vi "microplastic classifier front end.vi"() -> ()   [LabVIEW 2020]
panel:
  out "found processed and matched experimental data":bool
  out "Python Backend Log":string
  out "found mp library pickle":bool
  out "found python module":bool
  in  "Tab Control":enum32{"Experiment", "Library / Admin"}(tab)
  out "library entries":dbl
  out "Library Loaded":bool
  out "Min":dbl
  out "Max":dbl
  in  "Experimental Data Path":path=path "C:/Users/Matt/Desktop/Complete Lab View Programs/Microplastic Classifier V3/experimental data"
  in  "load  process match pickle exp data":bool
  in  "Export csv":bool
  in  "Export Images":bool
  in  "refresh library info":bool
  out "Boolean":bool
  out "saving pickle":bool
  in  "create pickle file from library":bool
  in  "error in (no error)":errorcluster
  out "error out 2":errorcluster
  in  "Raw Library Path":path=path "C:/Users/Matt/Desktop/Complete Lab View Programs/Microplastic Classifier V3/mp library"
  out "saved pickle":bool
  out "return value":i32
  in  "add test":bool
  in  "return path test":bool
  out "retunr path":string
  out "String":string
  out "Numeric":i32
  out "Numeric 2":i32
  out "Instructions":string
  in  "stop":bool
  # "Import Experimental Data\n    Step 1: Drag Experimental Data Folder into the box below\n    Step 2: Click the button to Load, Process & Match Data"
  # "Generate Reports:\n    -Step 3. Export .csv file or Export spectra images"
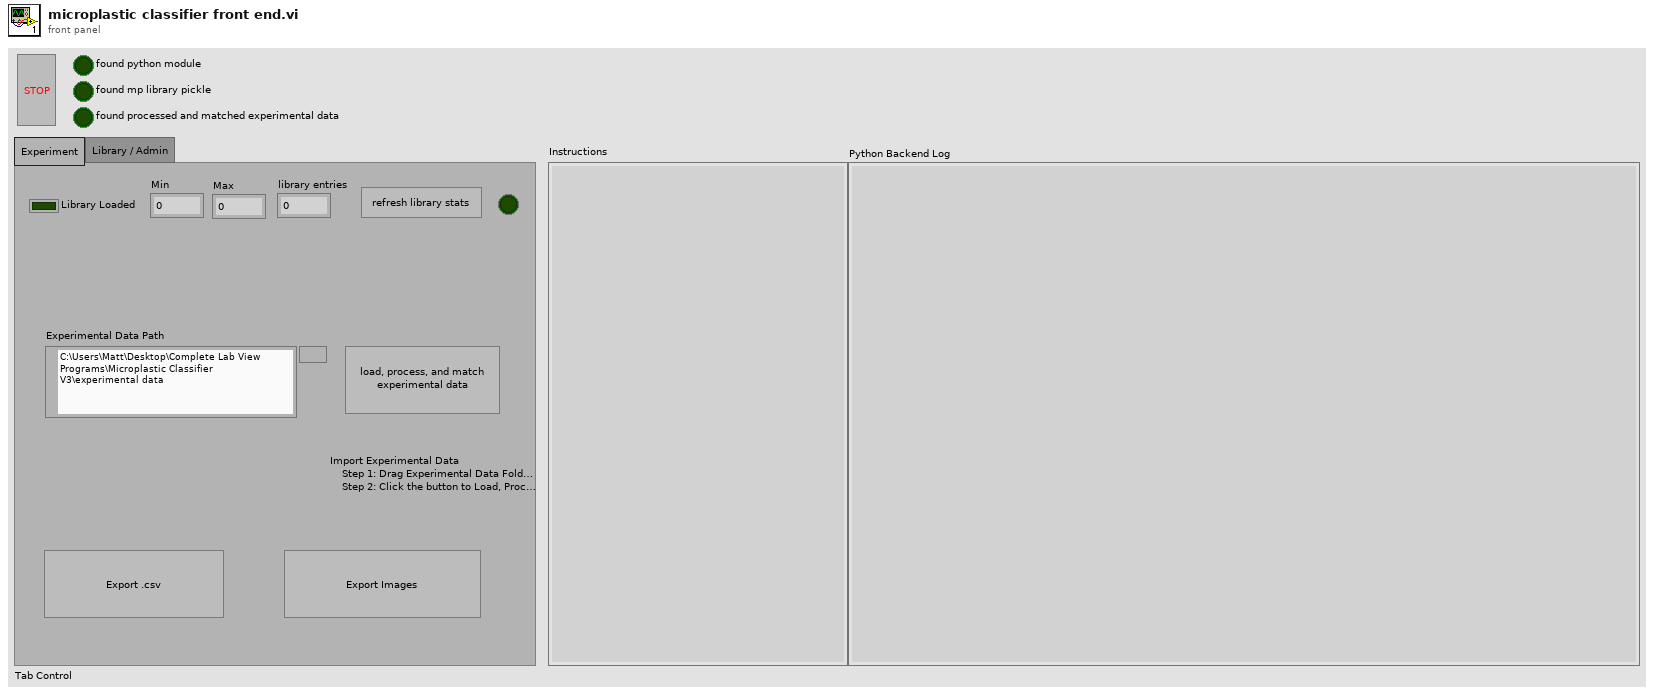
[diagram p1: front panel]
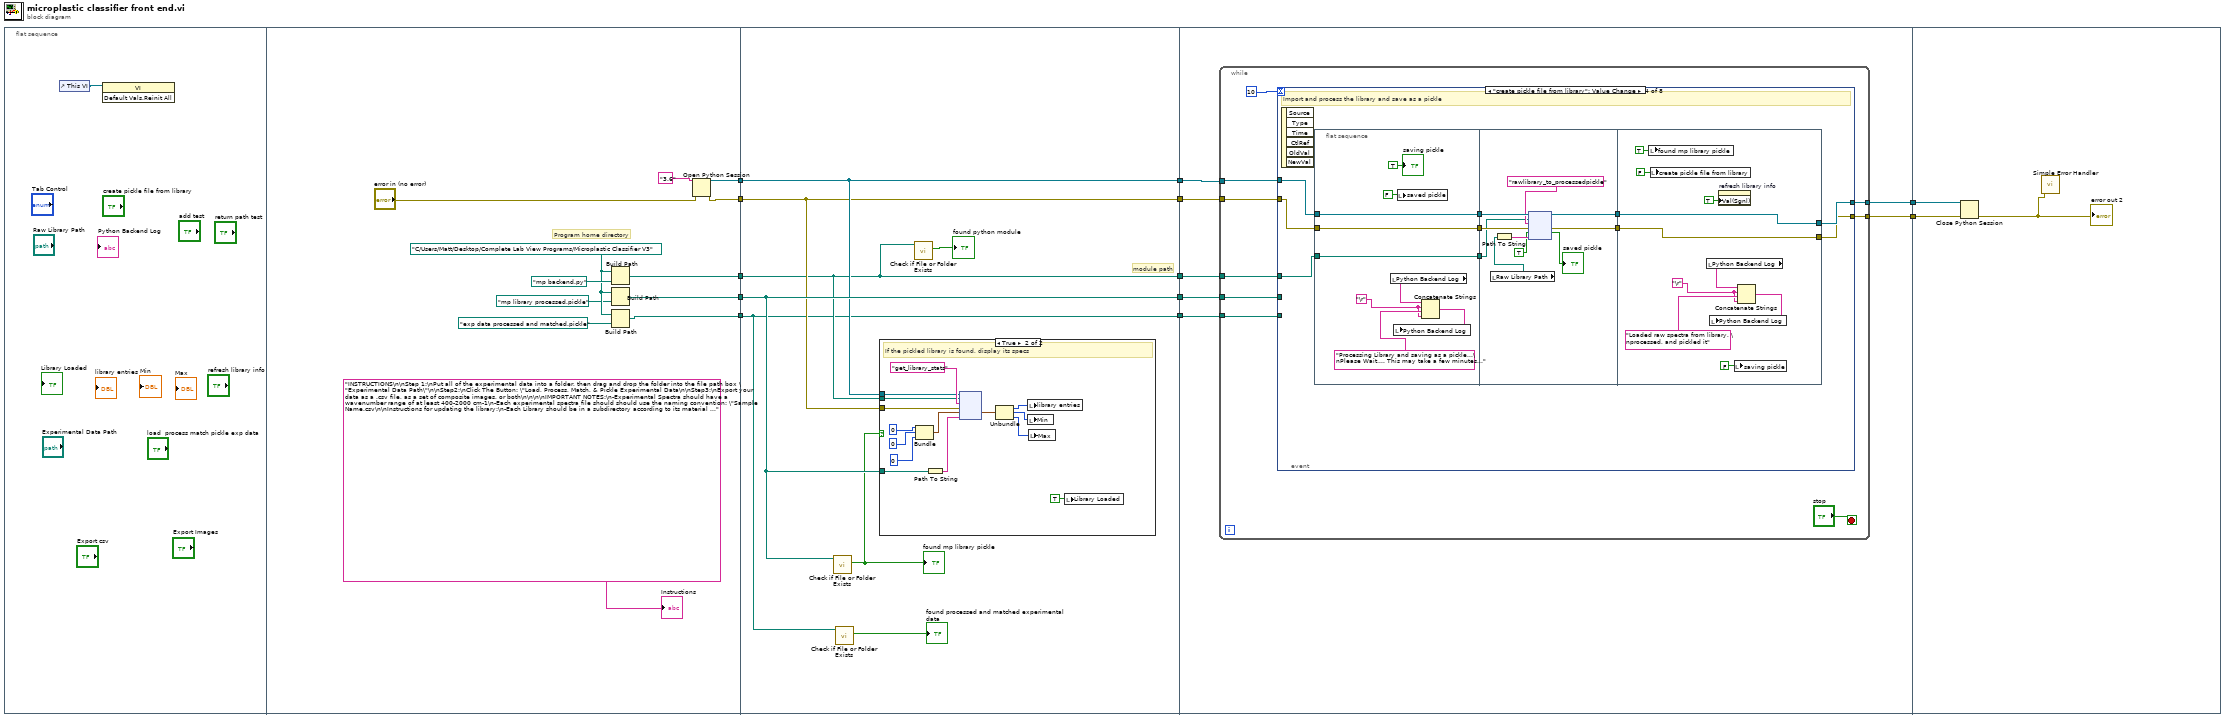
[diagram p0: block diagram]
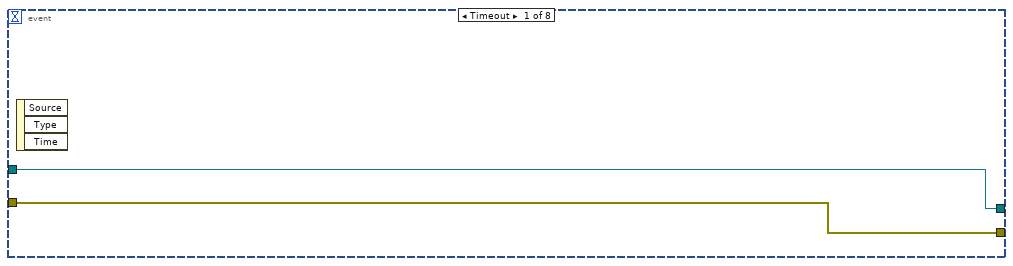
[diagram p3: hidden frame]
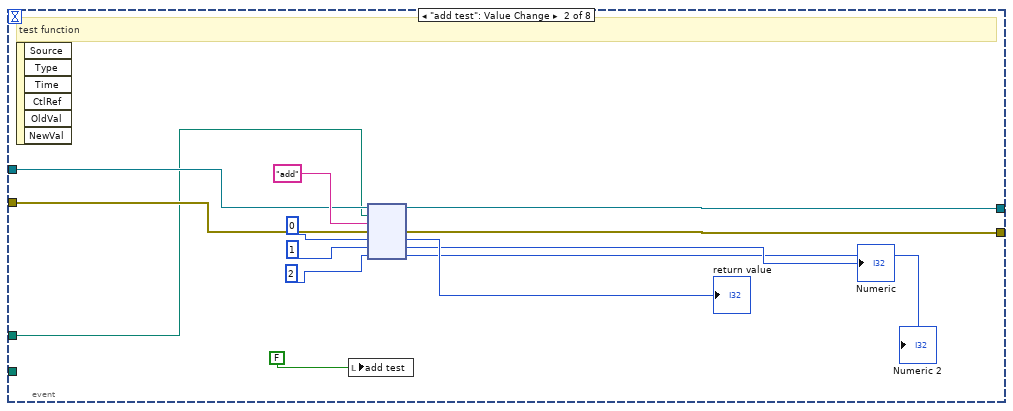
[diagram p4: hidden frame]
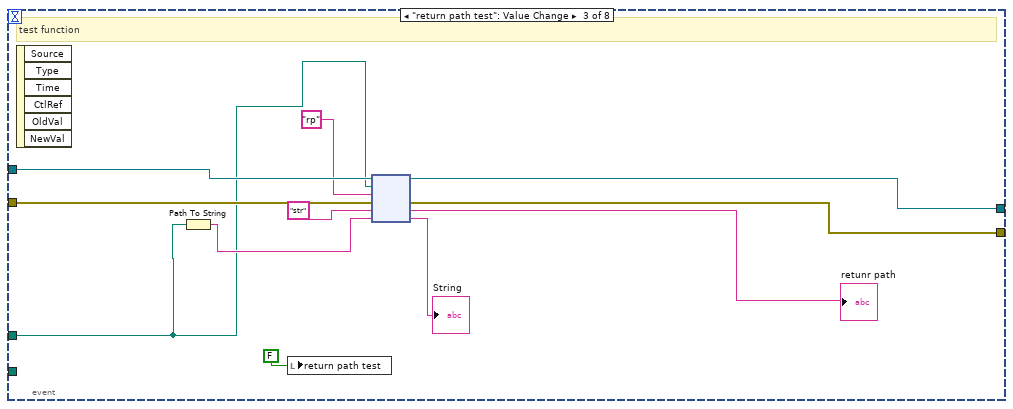
[diagram p5: hidden frame]
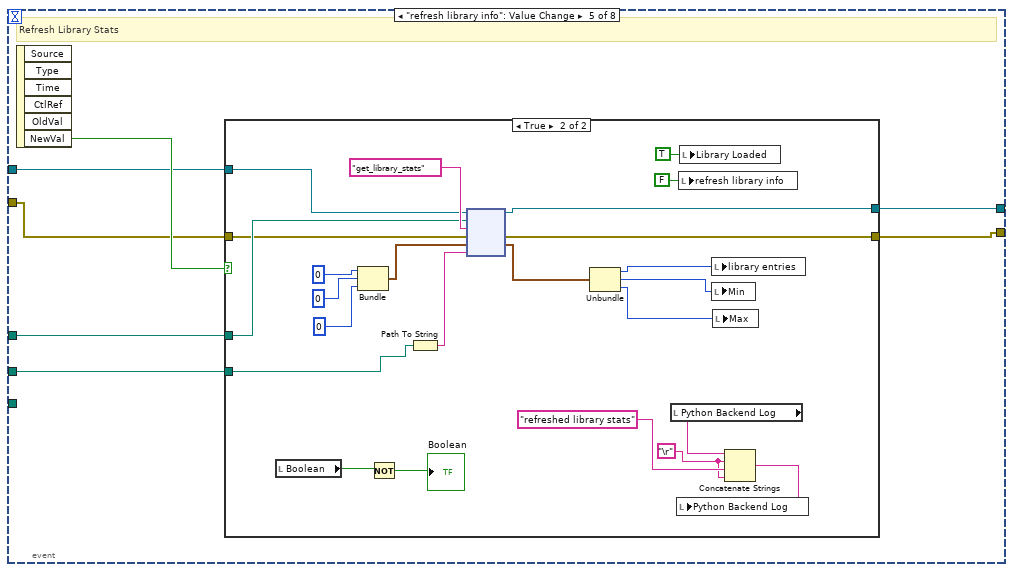
[diagram p6: hidden frame]
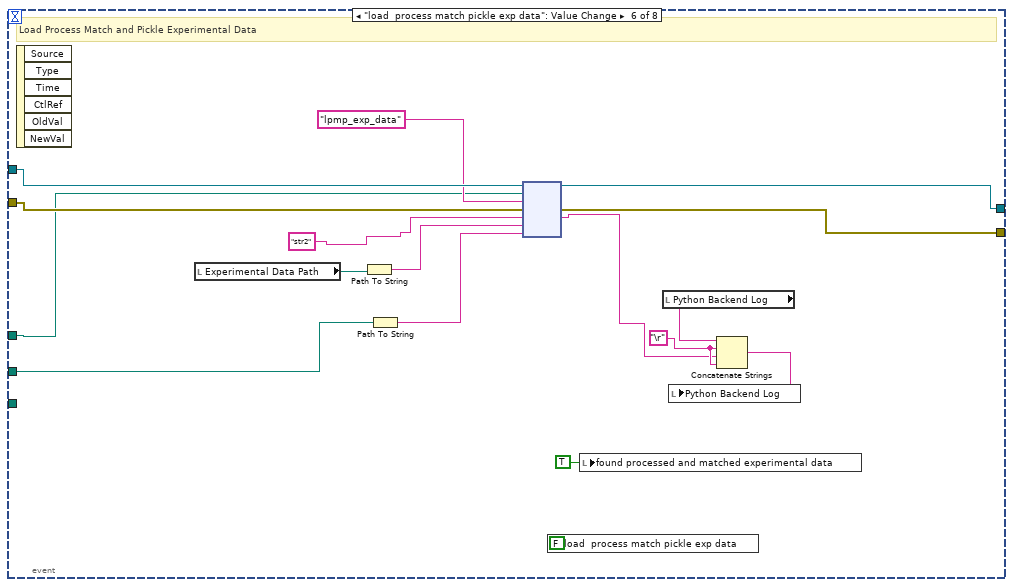
[diagram p8: hidden frame]
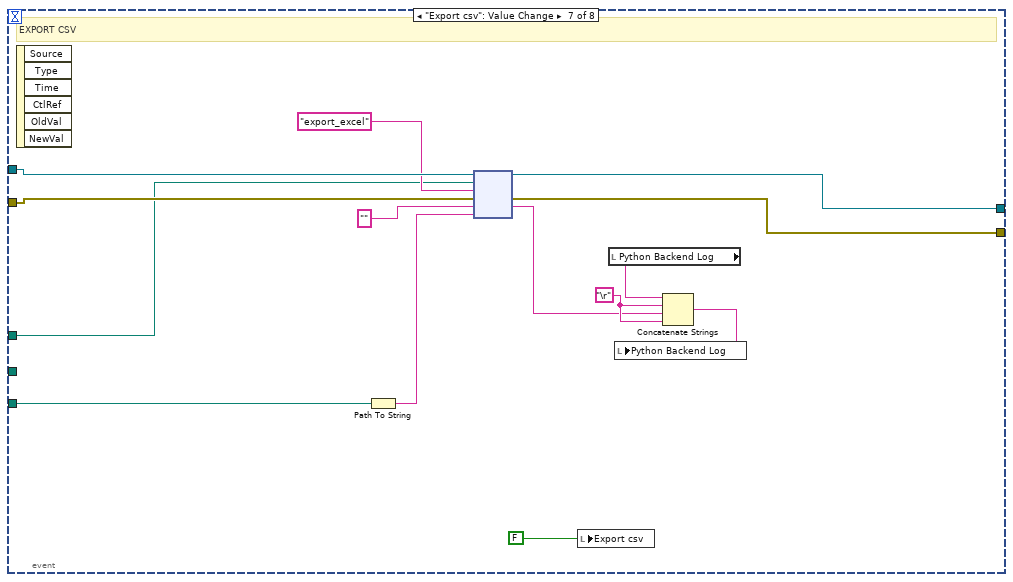
[diagram p9: hidden frame]
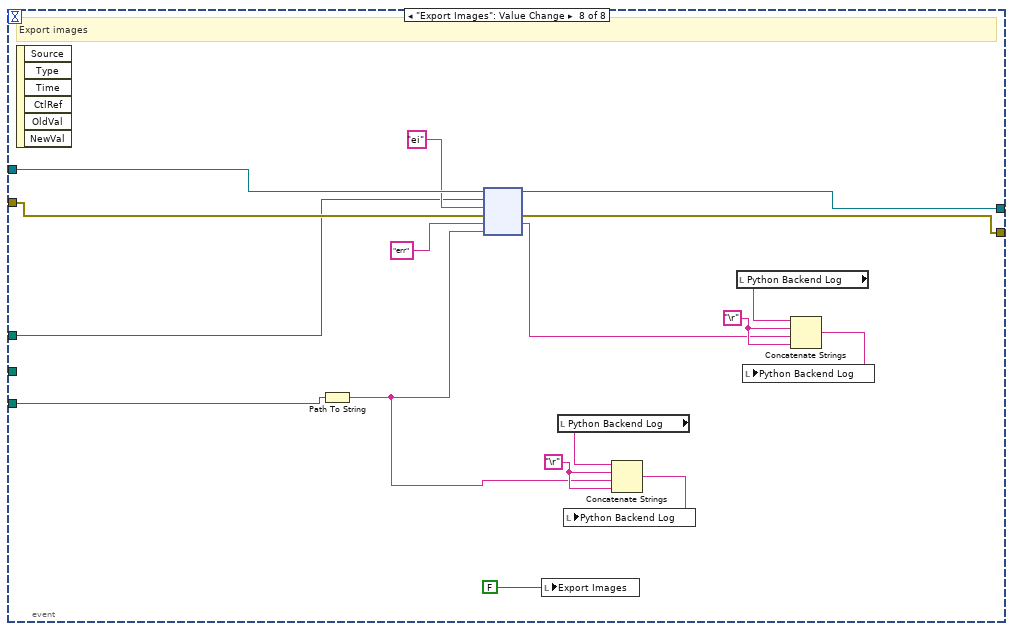
[diagram p10: hidden frame]
diagram:
  n1 = flat-sequence {
    tunnel: [w25] -> w10
    tunnel: [w24] -> w8
    tunnel: [w19] -> w6
    tunnel: [w17] -> w3
    tunnel: [w14] -> w1
    tunnel: w10 -> [w32]
    tunnel: [w32] -> w9
    tunnel: w8 -> [w31]
    tunnel: [w31] -> w7
    tunnel: w6 -> [w30]
    tunnel: [w30] -> w5
    tunnel: [w33] -> w4
    tunnel: w3 -> [w33]
    tunnel: [w26] -> w2
    tunnel: w1 -> [w26]
    tunnel: w9 -> [w55]
    tunnel: w7 -> [w54]
    tunnel: [w53] -> w12
    tunnel: [w52] -> w11
    tunnel: w5 -> [w51]
    tunnel: w4 -> [w50]
    tunnel: w2 -> [w49]
    tunnel: w12 -> [w213]
    tunnel: w11 -> [w212]
    frame #0 {
      n2 = control-ref of="This VI"() -> (w13:refnum<vi>)
      n3 = invoke class="VI" method="Default Vals.Reinit All"(reference=w13) -> ()  [unwired: 2 in, 3 out]
    }
    frame #1 {
      w18 = path "C:/Users/Matt/Desktop/Complete Lab View Programs/Microplastic Classifier V3" ("module path")
      # "Program home directory"
      n4 = Build Path(base path=w18, name or relative path=path "mp backend.py" ("module path")) -> (appended path=w19:path)
      n5 = Build Path(base path=w18, name or relative path=path "mp library processed.pickle" ("path")) -> (appended path=w17:path)
      n6 = Build Path(base path=w18, name or relative path=path "exp data processed and matched.pickle" ("path")) -> (appended path=w14:path)
      n7 = Open Python Session(python version="3.6" ("Python version"), 3:"error in (no error)") -> (session out=w25:refnum<k35>, error out=w24:errorcluster)  [unwired: 1 in]
      "Instructions" <- "INSTRUCTIONS\n\nStep 1:\nPut all of the experimental data into a folder, then drag and drop the folder into the file path box \"Experimental Data Path\"\n\nStep2:\nClick The Button: \"Load, Process, Match, & Pickle Experimental Data\n\nStep3:\nExport your data as a .csv file, as a set of composite images, or both\n\n\n\nIMPORTANT NOTES:\n-Experimental Spectra should have a wavenumber range of at least 400-2000 cm-1\n-Each experimental spectra file should should use the naming convention: \"Sample Name.csv\n\nInstructions for updating the library:\n-Each Library should be in a subdirectory according to its material classification\n-Library Entries should be at least 400-2000 cm-1\n-Specify the Library Folder by dragging the folder into the box: \"Library Path\"\n-Click the button \"Load, Process, & Pickle the Library\"\n-This does not need to be done if there is already a \"mp library.pickle\" file in the root folder" ("Instructions")
    }
    frame #2 {
      # "module path"
      n8 = call <vilib>:"Check if File or Folder Exists.vi"("path"=w33) -> ("file or folder exists?"=w29:bool)  [unwired: 8 in, 2 out]
      "found mp library pickle" <- w29
      n9 = call <vilib>:"Check if File or Folder Exists.vi"("path"=w26) -> ("file or folder exists?"=→"found processed and matched experimental data":bool)  [unwired: 8 in, 2 out]
      n10 = case shown="True" w29 {
        tunnel: w33 -> [_ w37]
        tunnel: w32 -> [_ w36]
        tunnel: w31 -> [_ w35]
        tunnel: w30 -> [_ w34]
        frame False {
        }
        frame True {
          # "If the pickled library is found, display its specs"
          n11 = Bundle(0, 0, 0) -> (w42:cluster{i32, i32, i32})  [unwired: 1 in]
          n12 = Path To String(path=w37) -> (string=w39:string)
          n13 = node(w36, w34, "get_library_stats" ("function name"), w35, w42, w39) -> (w43:cluster{i32, i32, i32})  [unwired: 1 in, 4 out]
          n14 = Unbundle(w43) -> (w47:i32, w46:i32, w45:i32)
          n15 = local write "library entries"(w47) -> ()
          n16 = local write "Min"(w46) -> ()
          n17 = local write "Max"(w45) -> ()
          n18 = local write "Library Loaded"(TRUE ("Library Loaded")) -> ()
        }
      }
      n19 = call <vilib>:"Check if File or Folder Exists.vi"("path"=w30) -> ("file or folder exists?"=→"found python module":bool)  [unwired: 8 in, 2 out]
    }
    frame #3 {
      n20 = while {
        tunnel: w55 -> [w62]
        tunnel: w54 -> [w61]
        tunnel: [w60] -> w53
        tunnel: [w59] -> w52
        tunnel: w51 -> [w58]
        tunnel: w50 -> [w57]
        tunnel: w49 -> [w56]
        stop <- "stop" stop-if-true
        n21 = event shown="[3] \"create pickle file from library\": Value Change" {
          selector: _ -> [_ _ _ _ _ _ _ _]
          dyn-events: _ -> [_ _ _ _ _ _ _ _]
          timeout: 10 -> [_ _ _ _ _ _ _ _]
          tunnel: w62 -> [w65 w73 w90 w100 w134 w179 w193 w210]
          tunnel: w61 -> [w66 w72 w87 w98 w131 w178 w192 w209]
          tunnel: [w65 w71 w89 w92 w133 w176 w190 w204] -> w60
          tunnel: [w66 w70 w88 w91 w132 w177 w191 w203] -> w59
          tunnel: w58 -> [_ w67 w80 w99 w135 w172 w185 w206]
          tunnel: w57 -> [_ _ _ _ w130 w171 _ _]
          tunnel: w56 -> [_ _ _ _ _ _ w186 w205]
          event Timeout {
            n22 = event-data() -> ()  [unwired: 1 in, 3 out]
          }
          event "add test": Value Change {
            # "test function"
            n23 = event-data() -> ()  [unwired: 1 in, 6 out]
            n24 = local write "add test"(FALSE ("export spectra match images")) -> ()
            n25 = node(w73, w67, "add" ("function name"), w72, 0, 1, 2) -> (w71:refnum<k35>, w70:errorcluster, →"return value":i32, →"Numeric":i32, →"Numeric 2":i32)  [unwired: 2 out]
          }
          event "return path test": Value Change {
            # "test function"
            n26 = event-data() -> ()  [unwired: 1 in, 6 out]
            n27 = Path To String(path=w80) -> (string=w83:string)
            n28 = local write "return path test"(FALSE ("return path test")) -> ()
            n29 = node(w90, w80, "rp" ("function name"), w87, "str" ("function name"), w83) -> (w89:refnum<k35>, w88:errorcluster, →"retunr path":string, →"String":string)  [unwired: 2 out]
          }
          event "create pickle file from library": Value Change {
            # "Import and process the library and save as a pickle"
            n30 = event-data() -> ()  [unwired: 1 in, 6 out]
            n31 = flat-sequence {
              tunnel: w98 -> [w107]
              tunnel: w99 -> [w108]
              tunnel: w100 -> [w109]
              tunnel: [w109] -> w95
              tunnel: [w108] -> w94
              tunnel: [w107] -> w93
              tunnel: [w114] -> w97
              tunnel: [w113] -> w96
              tunnel: w95 -> [w118]
              tunnel: w94 -> [w111]
              tunnel: w93 -> [w116]
              tunnel: w96 -> [w127]
              tunnel: w97 -> [w128]
              tunnel: [w128] -> w92
              tunnel: [w127] -> w91
              frame #0 {
                w101 = "\r"
                n32 = local read "Python Backend Log"() -> (w103:string)
                n33 = local write "saved pickle"(FALSE ("saved pickle")) -> ()
                n34 = Concatenate Strings(w103, w101, "Processing Library and saving as a pickle...\nPlease Wait.... This may take a few minutes..." ("function name"), w101) -> (w104:string)
                n35 = local write "Python Backend Log"(w104) -> ()
                "saving pickle" <- TRUE ("saving pickle")
              }
              frame #1 {
                n36 = local read "Raw Library Path"() -> (w112:path)
                n37 = Path To String(path=w112) -> (string=w119:string)
                n38 = node(w118, w111, "rawlibrary_to_processedpickle" ("function name"), w116, TRUE, w119) -> (w114:refnum<k35>, w113:errorcluster, →"saved pickle":bool)  [unwired: 1 in, 2 out]
              }
              frame #2 {
                w120 = "\r"
                n39 = local write "found mp library pickle"(TRUE ("found mp library pickle")) -> ()
                n40 = local write "create pickle file from library"(FALSE ("create pickle file from library")) -> ()
                n41 = local read "Python Backend Log"() -> (w125:string)
                n42 = property on="refresh library info" class="Bool (strict)"("Val(Sgnl)"=TRUE ("Value (Signaling)")) -> ()  [unwired: 2 in, 2 out]
                n43 = local write "saving pickle"(FALSE ("saving pickle")) -> ()
                n44 = Concatenate Strings(w125, w120, "Loaded raw spectra from library, \nprocessed, and pickled it", w120) -> (w126:string)
                n45 = local write "Python Backend Log"(w126) -> ()
              }
            }
          }
          event "refresh library info": Value Change {
            # "Refresh Library Stats"
            n46 = event-data() -> ("NewVal"=w136:bool)  [unwired: 1 in, 5 out]
            n47 = case shown="True" w136 {
              tunnel: w135 -> [_ w160]
              tunnel: w134 -> [w138 w159]
              tunnel: [w138 w158] -> w133
              tunnel: [w137 w157] -> w132
              tunnel: w131 -> [w137 w156]
              tunnel: w130 -> [_ w153]
              frame False {
              }
              frame True {
                w139 = "\r"
                n48 = local read "Boolean"() -> (w155:bool)
                n49 = Bundle(0, 0, 0) -> (w150:cluster{i32, i32, i32})  [unwired: 1 in]
                n50 = Not(x=w155) -> (.not. x?=→"Boolean":bool)
                n51 = Path To String(path=w153) -> (string=w143:string)
                n52 = node(w159, w160, "get_library_stats" ("function name"), w156, w150, w143) -> (w158:refnum<k35>, w157:errorcluster, w149:cluster{i32, i32, i32})  [unwired: 1 in, 2 out]
                n53 = Unbundle(w149) -> (w145:i32, w146:i32, w147:i32)
                n54 = local read "Python Backend Log"() -> (w141:string)
                n55 = local write "refresh library info"(FALSE ("refresh library info")) -> ()
                n56 = local write "Library Loaded"(TRUE ("Library Loaded")) -> ()
                n57 = local write "library entries"(w145) -> ()
                n58 = local write "Min"(w146) -> ()
                n59 = local write "Max"(w147) -> ()
                n60 = Concatenate Strings(w141, w139, "refreshed library stats" ("string"), w139) -> (w142:string)
                n61 = local write "Python Backend Log"(w142) -> ()
              }
            }
          }
          event "load  process match pickle exp data": Value Change {
            w165 = "\r"
            # "Load Process Match and Pickle Experimental Data"
            n62 = event-data() -> ()  [unwired: 1 in, 6 out]
            n63 = local read "Experimental Data Path"() -> (w174:path)
            n64 = Path To String(path=w174) -> (string=w173:string)
            n65 = Path To String(path=w171) -> (string=w170:string)
            n66 = node(w179, w172, "lpmp_exp_data" ("function name"), w178, "str2" ("function name"), w173, w170) -> (w176:refnum<k35>, w177:errorcluster, w164:string)  [unwired: 2 in, 2 out]
            n67 = local write "load  process match pickle exp data"(FALSE ("load and process exp data")) -> ()
            n68 = local write "found processed and matched experimental data"(TRUE ("found processed and matched experimental data")) -> ()
            n69 = local read "Python Backend Log"() -> (w166:string)
            n70 = Concatenate Strings(w166, w165, w164, w165) -> (w167:string)
            n71 = local write "Python Backend Log"(w167) -> ()
          }
          event "Export csv": Value Change {
            w181 = "\r"
            # "EXPORT CSV"
            n72 = event-data() -> ()  [unwired: 1 in, 6 out]
            n73 = Path To String(path=w186) -> (string=w187:string)
            n74 = node(w193, w185, "export_excel" ("function name"), w192, "" ("function name"), w187) -> (w190:refnum<k35>, w191:errorcluster, w180:string)  [unwired: 1 in, 2 out]
            n75 = local write "Export csv"(FALSE ("export matches as excel file")) -> ()
            n76 = local read "Python Backend Log"() -> (w182:string)
            n77 = Concatenate Strings(w182, w181, w180, w181) -> (w183:string)
            n78 = local write "Python Backend Log"(w183) -> ()
          }
          event "Export Images": Value Change {
            w198 = "\r"
            w199 = "\r"
            # "Export images"
            n79 = event-data() -> ()  [unwired: 1 in, 6 out]
            n80 = Path To String(path=w205) -> (string=w195:string)
            n81 = node(w210, w206, "ei" ("function name"), w209, "err" ("function name"), w195) -> (w204:refnum<k35>, w203:errorcluster, w194:string)  [unwired: 1 in, 2 out]
            n82 = local write "Export Images"(FALSE ("export matches as excel file")) -> ()
            n83 = local read "Python Backend Log"() -> (w197:string)
            n84 = Concatenate Strings(w197, w198, w195, w198) -> (w196:string)
            n85 = local write "Python Backend Log"(w196) -> ()
            n86 = local read "Python Backend Log"() -> (w200:string)
            n87 = Concatenate Strings(w200, w199, w194, w199) -> (w201:string)
            n88 = local write "Python Backend Log"(w201) -> ()
          }
        }
      }
    }
    frame #4 {
      n89 = Close Python Session(session in=w213, error in=w212) -> (11:w211:errorcluster)
      "error out 2" <- w211
      n90 = call <vilib>:"Simple Error Handler.vi"("error in (no error)"=w211) -> ()  [unwired: 4 in, 5 out]
    }
  }
